vi "PDP uWaveFreq= Message.vi"(0 "uWave Freq":dbl format="%.3f") -> ()   [LabVIEW 2019]
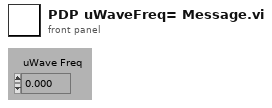
[diagram p1: front panel]
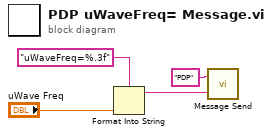
[diagram p0: block diagram]
diagram:
  n1 = Format Into String(format string="uWaveFreq=%.3f" ("Format String"), "uWave Freq") -> (resulting string=w1:string)  [unwired: 2 in, 1 out]
  n2 = call "Message Send.vi"("Message"=w1, "Destination"="PDP") -> ()
